vi "AB_820_850_Project_Source_DependencyNode.vi"(6 "dataForPrevious":T2, 7 "action":T1, 8 "error in (no error)":errorcluster, 10 "data in":T6, 11 "buildObject in":T7) -> (0 "error out":errorcluster, 2 "data out":T6, 3 "buildObject out":T7)   [LabVIEW 2020]
doc: "Reads and writes the data to the object property bag."
uses:
  <resource>/Framework/Providers/API/ItemRef.ctl
  <vilib>/AppBuilder/AB_Source_Inclusion.ctl
  <vilib>/AppBuilder/RW_Project/AB_RW_Project_Source_Data_for_Previous.ctl
  <vilib>/AppBuilder/AB_BuildType.ctl
  <vilib>/Utility/lvfile.llb/LVFileType.ctl
  <vilib>/AppBuilder/RW_Project/AB_RW_Project_PropBag_Action.ctl
  <vilib>/Utility/lvfile.llb/NI_FileType.lvlib
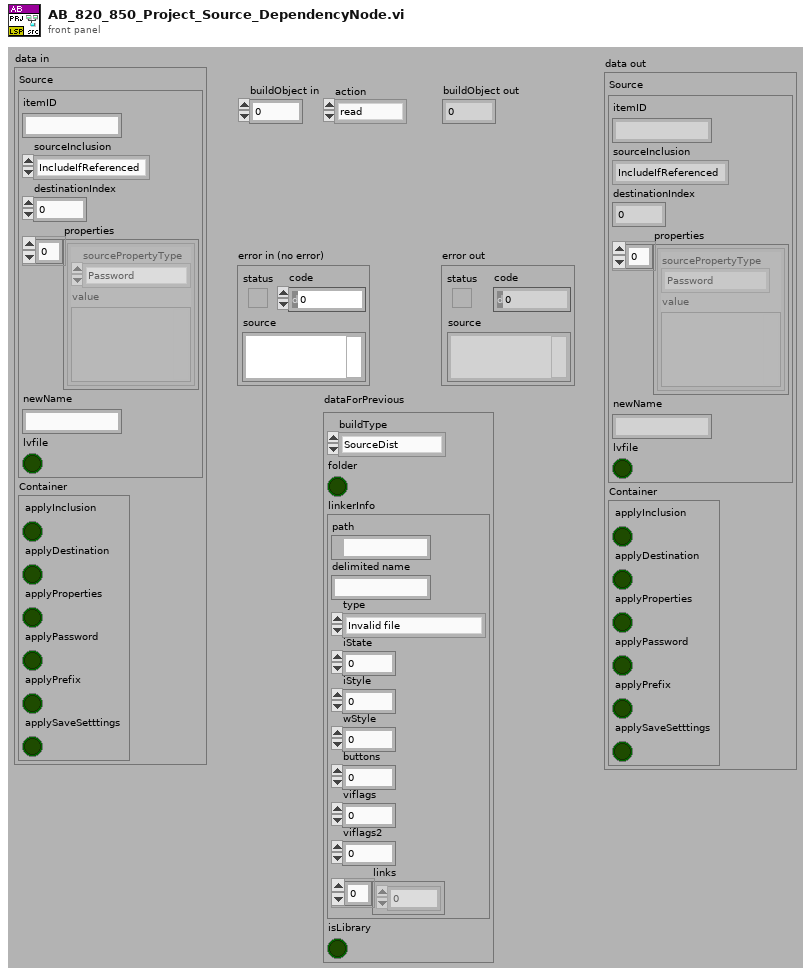
[diagram p1: front panel]
types:
  T1 = typedef "AB_RW_Project_PropBag_Action.ctl" = enum16{"read", "write", "clear", "readPrevious", "writePrevious", "clearPrevious"}
  T2 = typedef "AB_RW_Project_Source_Data_for_Previous.ctl" = cluster{"buildType":T3, "folder":bool, "linkerInfo":cluster{"path":path, "delimited name":string, "type":T4, "iState":u32, "iStyle":u16, "wStyle":u16, "buttons":u16, "viflags":u32, "viflags2":u32, "links":u32[]}, "isLibrary":bool}
  T3 = typedef "AB_BuildType.ctl" = enum16{"SourceDist", "EXE", "DLL", "RTExe"}
  T4 = typedef "NI_FileType.lvlib/LVFileType.ctl" = enum32{"Invalid file", "Unknown type", "Instrument", "Control", "Polymorphic VI", "Project", "Library", "LVClass", "XControl", "XNode", "Shared library", ".NET assembly", "ActiveX interface", "CIN", "Run-time menu", "Palette menu", "Help file", "LLB", "XNode Edit Dependency", "Class Private Data Control", "Statechart", "MathScript .m file", "Ladder Diagram", "LVLibp", "XNode Build Dependency"}
  T5 = typedef "AB_Source_Inclusion.ctl" = enum16{"IncludeIfReferenced", "Include", "Exclude", "TopLevel"}
  T6 = cluster{"Source":cluster{"itemID":string, "sourceInclusion":T5, "destinationIndex":i32, "properties":cluster{"sourcePropertyType":enum16{"Remove block diagram", "Remove front panel", "Password", "Window has title bar", "Show menu bar", "Show vertical scroll bar", "Show horizontal scroll bar", "Show toolbar", "Show Abort button", "Show fp when called", "Window behavior", "Allow user to close window", "Window run-time position", "Run when opened", "Allow debugging", "Auto error handling"}, "value":variant}[], "newName":string, "lvfile":bool}, "Container":cluster{"applyInclusion":bool, "applyDestination":bool, "applyProperties":bool, "applyPassword":bool, "applyPrefix":bool, "applySaveSetttings":bool}}
  T7 = typedef "ItemRef.ctl" = u64
  T8 = cluster{"sourcePropertyType":enum16{"Remove block diagram", "Remove front panel", "Password", "Window has title bar", "Show menu bar", "Show vertical scroll bar", "Show horizontal scroll bar", "Show toolbar", "Show Abort button", "Show fp when called", "Window behavior", "Allow user to close window", "Window run-time position", "Run when opened", "Allow debugging", "Auto error handling"}, "value":variant}
  T9 = enum16{"Remove block diagram", "Remove front panel", "Password", "Window has title bar", "Show menu bar", "Show vertical scroll bar", "Show horizontal scroll bar", "Show toolbar", "Show Abort button", "Show fp when called", "Window behavior", "Allow user to close window", "Window run-time position", "Run when opened", "Allow debugging", "Auto error handling"}
  T10 = cluster{"pre-2010 typedef (disconnected)":enum16{"Remove block diagram", "Remove front panel", "Password", "Window has title bar", "Show menu bar", "Show vertical scroll bar", "Show horizontal scroll bar", "Show toolbar", "Show Abort button", "Show fp when called", "Window behavior", "Allow user to close window", "Window run-time position", "Run when opened", "Allow debugging", "Auto error handling"}, "Value":string}
  T11 = cluster{"sourcePropertyType":enum16{"Remove block diagram", "Remove front panel", "Password", "Window has title bar", "Show menu bar", "Show vertical scroll bar", "Show horizontal scroll bar", "Show toolbar", "Show Abort button", "Show fp when called", "Window behavior", "Allow user to close window", "Window run-time position", "Run when opened", "Allow debugging", "Auto error handling"}, "value":variant}[]
  T12 = cluster{"pre-2010 typedef (disconnected)":enum16{"Remove block diagram", "Remove front panel", "Password", "Window has title bar", "Show menu bar", "Show vertical scroll bar", "Show horizontal scroll bar", "Show toolbar", "Show Abort button", "Show fp when called", "Window behavior", "Allow user to close window", "Window run-time position", "Run when opened", "Allow debugging", "Auto error handling"}, string}
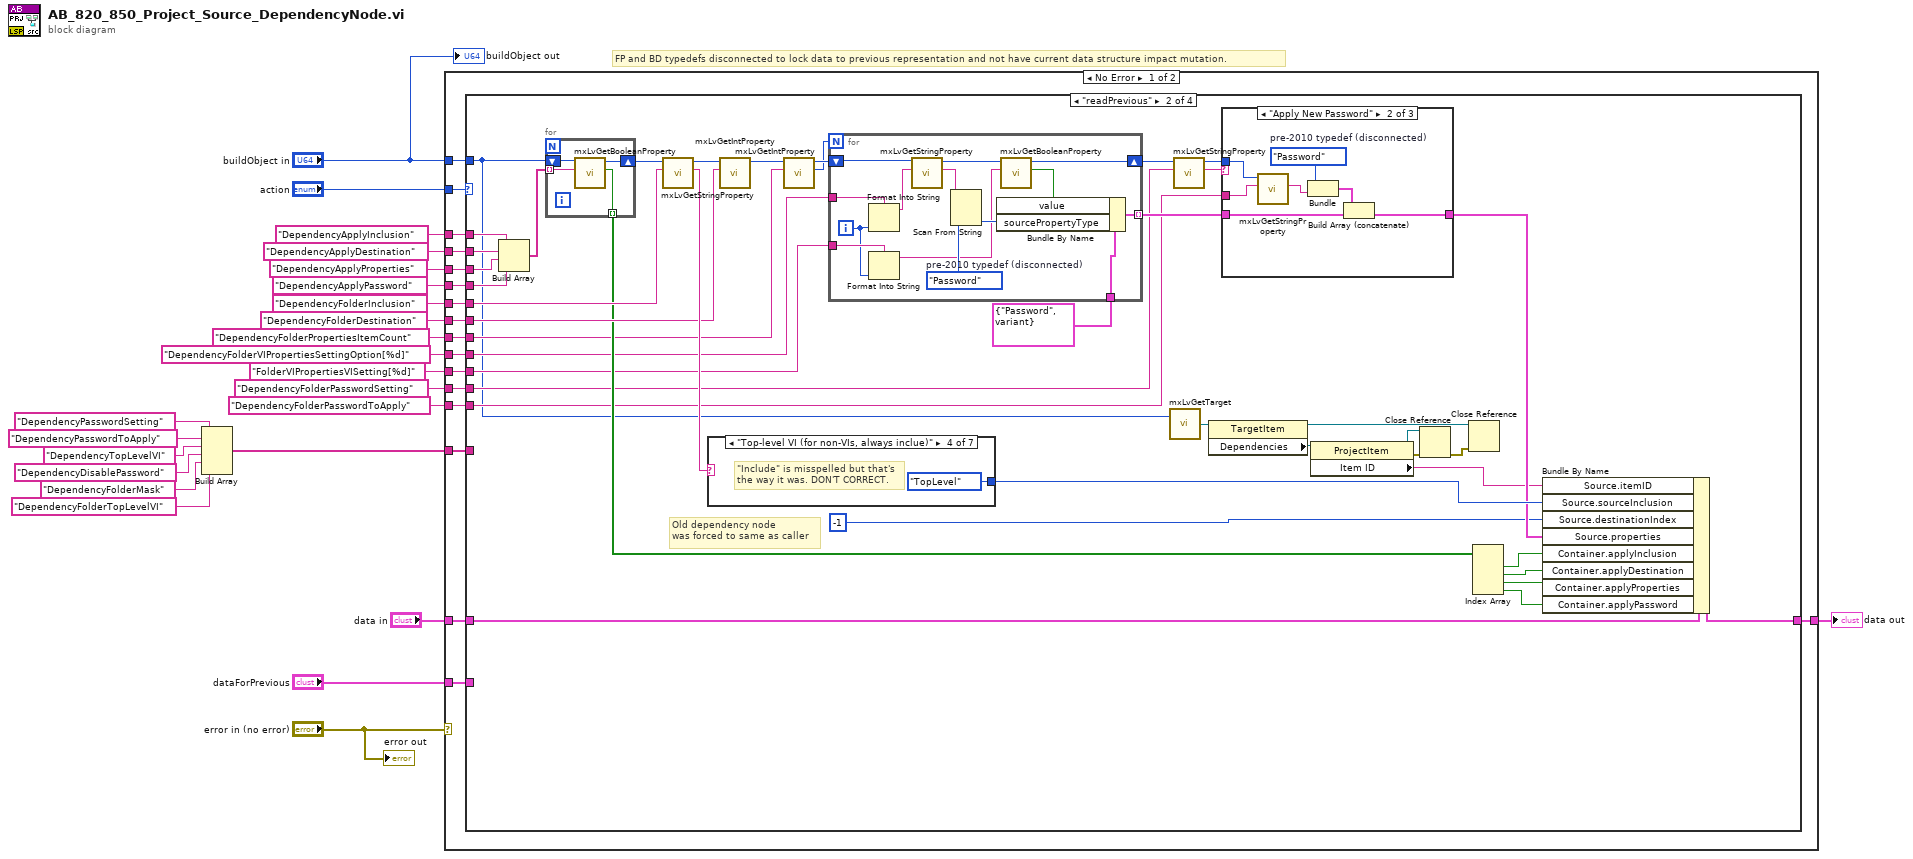
[diagram p0: block diagram]
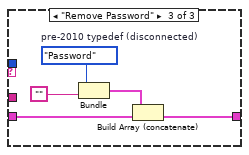
[diagram p4: hidden frame]
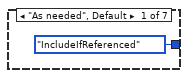
[diagram p5: hidden frame]
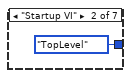
[diagram p6: hidden frame]
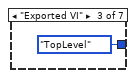
[diagram p7: hidden frame]
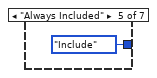
[diagram p8: hidden frame]
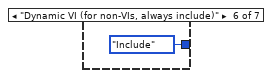
[diagram p9: hidden frame]
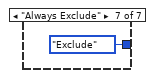
[diagram p10: hidden frame]
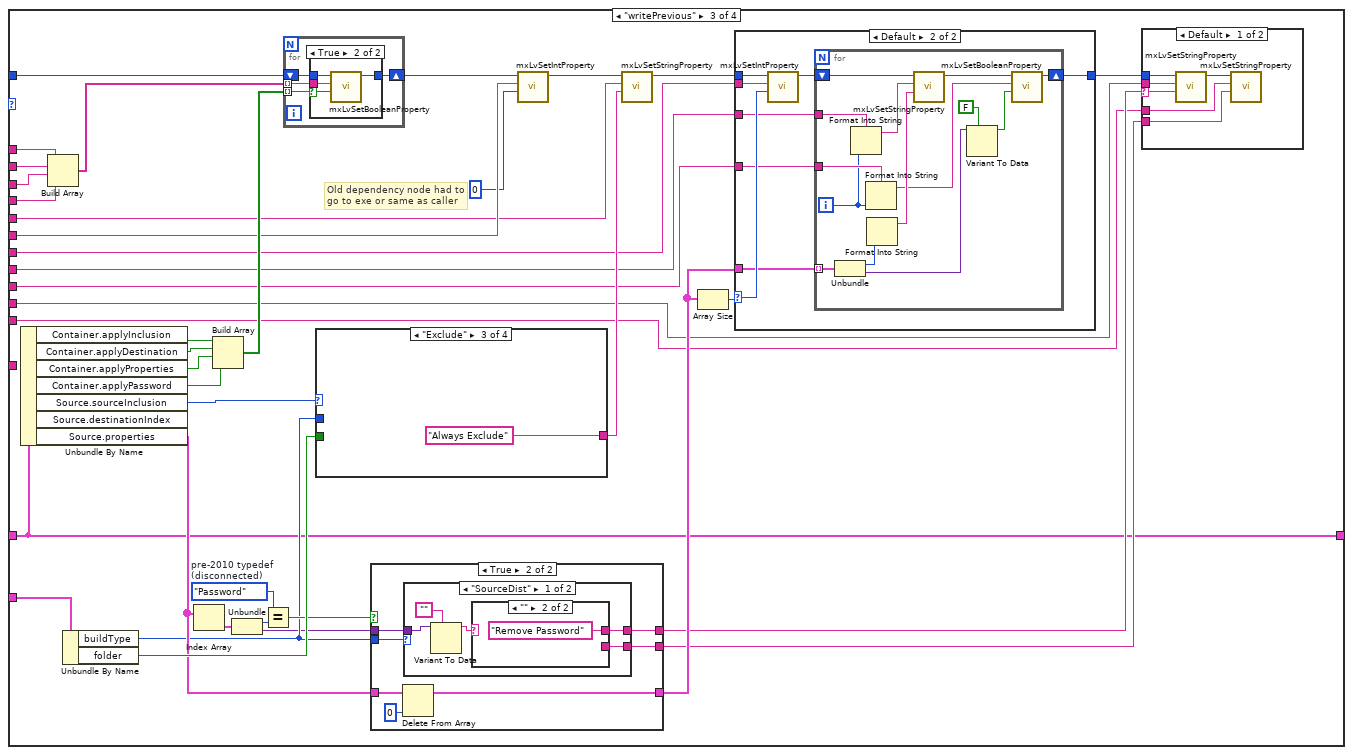
[diagram p11: hidden frame]
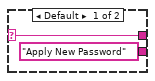
[diagram p15: hidden frame]
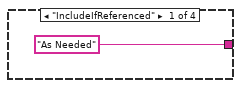
[diagram p17: hidden frame]
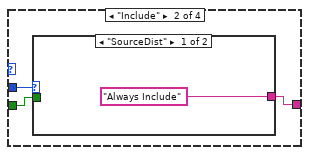
[diagram p18: hidden frame]
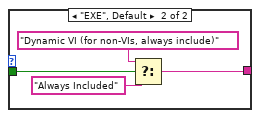
[diagram p19: hidden frame]
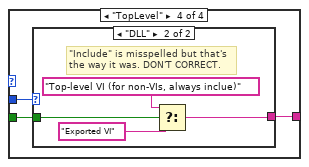
[diagram p20: hidden frame]
diagram:
  # "FP and BD typedefs disconnected to lock data to previous representation and not have current data structure impact mutation."
  n1 = Build Array("DependencyPasswordSetting", "DependencyPasswordToApply", "DependencyTopLevelVI", "DependencyDisablePassword", "DependencyFolderMask", "DependencyFolderTopLevelVI") -> (w2:string[])
  n2 = case shown="No Error" "error in (no error)" {
    tunnel: "buildObject in" -> [w28 _]
    tunnel: "DependencyApplyInclusion" -> [w37 _]
    tunnel: "DependencyFolderInclusion" -> [w41 _]
    tunnel: "DependencyApplyDestination" -> [w38 _]
    tunnel: "DependencyFolderDestination" -> [w40 _]
    tunnel: "DependencyFolderPropertiesItemCount" -> [w34 _]
    tunnel: "DependencyApplyProperties" -> [w36 _]
    tunnel: "data in" -> [w39 w264]
    tunnel: "DependencyApplyPassword" -> [w35 _]
    tunnel: "DependencyFolderVIPropertiesSettingOption[%d]" -> [w33 _]
    tunnel: "FolderVIPropertiesVISetting[%d]" -> [w32 _]
    tunnel: "DependencyFolderPasswordToApply" -> [w31 _]
    tunnel: "DependencyFolderPasswordSetting" -> [w30 _]
    tunnel: [w29 w264] -> w11
    tunnel: "action" -> [w27 _]
    tunnel: "dataForPrevious" -> [w26 _]
    tunnel: w2 -> [w25 _]
    frame No Error {
      n3 = case shown="\"readPrevious\"" w27 {
        tunnel: w41 -> [_ w81 w129 w248]
        tunnel: w40 -> [_ w80 w130 w247]
        tunnel: w39 -> [w42 w79 w123 w253]
        tunnel: w38 -> [_ w78 w140 w251]
        tunnel: w37 -> [_ w77 w141 w252]
        tunnel: w36 -> [_ w76 w139 w250]
        tunnel: w35 -> [_ w75 w138 w249]
        tunnel: w34 -> [_ w58 w128 w244]
        tunnel: w33 -> [_ w57 w127 w242]
        tunnel: w32 -> [_ w56 w126 w241]
        tunnel: w31 -> [_ w55 w124 w239]
        tunnel: w30 -> [_ w54 w125 w240]
        tunnel: [w42 w52 w123 w253] -> w29
        tunnel: w28 -> [_ w51 w142 w246]
        tunnel: w26 -> [_ _ w132 _]
        tunnel: w25 -> [_ _ _ w236]
        frame Default {
        }
        frame "readPrevious" {
          # "Old dependency node\nwas forced to same as caller"
          n4 = Build Array(w77, w78, w76, w75) -> (w74:string[])
          n5 = for {
            tunnel: w74 -> [w112] mode=indexing
            shift-right: [w114] -> w83
            shift-left: w51 -> [w113]
            tunnel: [w111] -> w73 mode=indexing
            n6 = call <resource>:"mxLvGetBooleanProperty.vi"("Tag"=w112, "Item"=w113) -> ("Value"=w111:bool, "Item"=w114:T7)  [unwired: 1 in, 7 out]
          }
          n7 = call <resource>:"mxLvGetStringProperty.vi"("Tag"=w81, "Item"=w83) -> ("Value"=w82:string, "Item"=w68:T7)  [unwired: 1 in, 7 out]
          n8 = case shown="\"Top-level VI (for non-VIs, always inclue)\"" w82 {
            tunnel: [AB_Source_Inclusion."IncludeIfReferenced" ("sourceInfo.sourceInclusion") AB_Source_Inclusion."TopLevel" ("sourceInfo.sourceInclusion") AB_Source_Inclusion."TopLevel" ("sourceInfo.sourceInclusion") AB_Source_Inclusion."TopLevel" ("sourceInfo.sourceInclusion") AB_Source_Inclusion."Include" ("sourceInfo.sourceInclusion") AB_Source_Inclusion."Include" ("sourceInfo.sourceInclusion") AB_Source_Inclusion."Exclude" ("sourceInfo.sourceInclusion")] -> w67
            frame "As needed", Default {
            }
            frame "Startup VI" {
            }
            frame "Exported VI" {
            }
            frame "Top-level VI (for non-VIs, always inclue)" {
              # "\"Include\" is misspelled but that's the way it was. DON'T CORRECT."
            }
            frame "Always Included" {
            }
            frame "Dynamic VI (for non-VIs, always include)" {
            }
            frame "Always Exclude" {
            }
          }
          n9 = call <resource>:"mxLvGetIntProperty.vi"("Tag"=w80, "Item"=w68) -> ("Item"=w59:T7)  [unwired: 1 in, 8 out]
          n10 = call <resource>:"mxLvGetIntProperty.vi"("Tag"=w58, "Item"=w59) -> ("Value"=w60:i32, "Item"=w66:T7)  [unwired: 1 in, 7 out]
          n11 = for {
            N: w60 -> [_]
            tunnel: T8 {"sourcePropertyType"=enum."Password", "value"=variant} ("fileProperties") -> [w108]
            tunnel: [w107] -> w65 mode=indexing
            tunnel: w57 -> [w101]
            tunnel: w56 -> [w98]
            shift-right: [w102] -> w62
            shift-left: w66 -> [w110]
            i -> [w97]
            w104 = T9."Password"  # pre-2010 typedef (disconnected)
            n12 = Format Into String(format string=w101, w97) -> (resulting string=w100:string)  [unwired: 2 in, 1 out]
            n13 = Format Into String(format string=w98, w97) -> (resulting string=w99:string)  [unwired: 2 in, 1 out]
            n14 = call <resource>:"mxLvGetStringProperty.vi"("Tag"=w100, "Item"=w110) -> ("Value"=w105:string, "Item"=w109:T7)  [unwired: 1 in, 7 out]
            n15 = Scan From String(input string=w105, default 1=w104) -> (output 1=w103:T9)  [unwired: 3 in, 3 out]
            n16 = call <resource>:"mxLvGetBooleanProperty.vi"("Tag"=w99, "Item"=w109) -> ("Value"=w106:bool, "Item"=w102:T7)  [unwired: 1 in, 7 out]
            n17 = Bundle By Name(cluster=w108, "value"=w106, "sourcePropertyType"=w103) -> (w107:T8)
          }
          n18 = call <resource>:"mxLvGetTarget.vi"("Item"=w51) -> ("Target"=w50:refnum<vi>)  [unwired: 1 in, 2 out]
          n19 = call <resource>:"mxLvGetStringProperty.vi"("Tag"=w54, "Item"=w62) -> ("Value"=w63:string, "Item"=w64:T7)  [unwired: 1 in, 7 out]
          n20 = property class="TargetItem"(reference=w50) -> (reference out=w43:refnum<vi>, "Dependencies"=w49:refnum<vi>)  [unwired: 1 in, 1 out]
          n21 = case shown="\"Apply New Password\"" w63 {
            tunnel: w64 -> [_ w91 _]
            tunnel: w55 -> [_ w90 _]
            tunnel: w65 -> [w84 w89 w96]
            tunnel: [w84 w85 w93] -> w53
            frame "No Password Change", Default {
            }
            frame "Apply New Password" {
              w88 = T9."Password"  # pre-2010 typedef (disconnected)
              n22 = call <resource>:"mxLvGetStringProperty.vi"("Tag"=w90, "Item"=w91) -> ("Value"=w87:string)  [unwired: 1 in, 8 out]
              n23 = Bundle("pre-2010 typedef (disconnected)"=w88, "Value"=w87) -> (w86:T10)  [unwired: 1 out]
              n24 = Build Array (concatenate)(w86, w89) -> (w85:T11)
            }
            frame "Remove Password" {
              w95 = T9."Password"  # pre-2010 typedef (disconnected)
              n25 = Bundle("pre-2010 typedef (disconnected)"=w95, "") -> (w94:T12)  [unwired: 1 out]
              n26 = Build Array (concatenate)(w94, w96) -> (w93:T11)
            }
          }
          n27 = property class="ProjectItem"(reference=w49) -> (reference out=w46:refnum<vi>, error out=w45:errorcluster, "Item ID"=w48:string)  [unwired: 1 in]
          n28 = Close Reference(reference=w46, error in (no error)=w45) -> (error out=w44:errorcluster)
          n29 = Close Reference(reference=w43, error in (no error)=w44) -> ()  [unwired: 1 out]
          n30 = Index Array(array=w73) -> (element #1=w72:bool, element #2=w71:bool, element #3=w70:bool, element #4=w69:bool)  [unwired: 4 in]
          n31 = Bundle By Name(cluster=w79, "Source.itemID"=w48, "Source.sourceInclusion"=w67, "Source.destinationIndex"=-1, "Source.properties"=w53, "Container.applyInclusion"=w72, "Container.applyDestination"=w71, "Container.applyProperties"=w70, "Container.applyPassword"=w69) -> (w52:T6)
        }
        frame "writePrevious" {
          w154 = T9."Password"  # pre-2010 typedef (disconnected)
          # "Old dependency node had to go to exe or same as caller"
          n32 = Unbundle By Name(w123) -> ("Container.applyInclusion"=w137:bool, "Container.applyDestination"=w136:bool, "Container.applyProperties"=w135:bool, "Container.applyPassword"=w134:bool, "Source.sourceInclusion"=w159:T5, "Source.properties"=w152:T11)  [unwired: 1 out]
          n33 = Build Array(w141, w140, w139, w138) -> (w143:string[])
          n34 = Unbundle By Name(w132) -> ("buildType"=w151:T3, "folder"=w158:bool)
          n35 = Index Array(array=w152) -> (element=w156:T8)  [unwired: 1 in]
          n36 = Build Array(w137, w136, w135, w134) -> (w133:bool[])
          n37 = Unbundle(w156) -> ("sourcePropertyType"=w155:T9, "value"=w150:variant)
          n38 = Equal?(x=w154, y=w155) -> (x = y?=w153:bool)
          n39 = for {
            tunnel: w143 -> [w162] mode=indexing
            shift-right: [w163] -> w131
            shift-left: w142 -> [w164]
            tunnel: w133 -> [w161] mode=indexing
            n40 = case shown="True" w161 {
              selector: w161 -> [_ w166]
              tunnel: w164 -> [w165 w169]
              tunnel: [w165 w168] -> w163
              tunnel: w162 -> [_ w167]
              frame False {
              }
              frame True {
                n41 = call <resource>:"mxLvSetBooleanProperty.vi"("Value (F)"=w166, "Tag"=w167, "Item"=w169) -> ("Item"=w168:T7)  [unwired: 2 in, 6 out]
              }
            }
          }
          n42 = case shown="\"Exclude\"" w159 {
            tunnel: w151 -> [_ w195 _ w204]
            tunnel: w158 -> [_ w194 _ w203]
            tunnel: ["As Needed" w193 "Always Exclude" w202] -> w157
            frame "IncludeIfReferenced" {
            }
            frame "Include" {
              n43 = case shown="\"SourceDist\"" w195 {
                tunnel: w194 -> [_ w200]
                tunnel: ["Always Include" w197] -> w193
                frame "SourceDist" {
                }
                frame "EXE", Default {
                  n44 = Select(t="Dynamic VI (for non-VIs, always include)", s=w200, f="Always Included") -> (s? t:f=w197:string)
                }
              }
            }
            frame "Exclude" {
            }
            frame "TopLevel" {
              n45 = case shown="\"DLL\"" w204 {
                tunnel: w203 -> [w208 w212]
                tunnel: [w205 w209] -> w202
                frame "EXE", Default {
                  # "\"Include\" is misspelled but that's the way it was. DON'T CORRECT."
                  n46 = Select(t="Top-level VI (for non-VIs, always inclue)", s=w208, f="Startup VI") -> (s? t:f=w205:string)
                }
                frame "DLL" {
                  # "\"Include\" is misspelled but that's the way it was. DON'T CORRECT."
                  n47 = Select(t="Top-level VI (for non-VIs, always inclue)", s=w212, f="Exported VI") -> (s? t:f=w209:string)
                }
              }
            }
          }
          n48 = case shown="True" w153 {
            tunnel: w152 -> [w176 w183]
            tunnel: [w176 w181] -> w149
            tunnel: w151 -> [_ w180]
            tunnel: w150 -> [_ w179]
            tunnel: [_ w178] -> w146
            tunnel: [_ w177] -> w144
            frame False {
            }
            frame True {
              n49 = Delete From Array(array=w183, index=0) -> (array with subset deleted=w181:T11)  [unwired: 1 in, 1 out]
              n50 = case shown="\"SourceDist\"" w180 {
                tunnel: w179 -> [w187 _]
                tunnel: [w185 _] -> w178
                tunnel: [w184 _] -> w177
                frame "SourceDist" {
                  n51 = Variant To Data(type="", Variant=w187) -> (data=w186:string)  [unwired: 1 in, 1 out]
                  n52 = case shown="\"\"" w186 {
                    selector: w186 -> [w190 _]
                    tunnel: [w190 "Remove Password"] -> w185
                    tunnel: ["Apply New Password" _] -> w184
                    frame Default {
                    }
                    frame "" {
                    }
                  }
                }
                frame Default {
                }
              }
            }
          }
          n53 = call <resource>:"mxLvSetIntProperty.vi"("Value (0)"=0, "Tag"=w130, "Item"=w131) -> ("Item"=w148:T7)  [unwired: 2 in, 6 out]
          n54 = call <resource>:"mxLvSetStringProperty.vi"("Value (\"\")"=w157, "Tag"=w129, "Item"=w148) -> ("Item"=w147:T7)  [unwired: 2 in, 6 out]
          n55 = Array Size(array=w149) -> (size(s)=w160:i32)
          n56 = case shown="Default" w160 {
            selector: w160 -> [_ w219]
            tunnel: w149 -> [_ w217]
            tunnel: w128 -> [_ w221]
            tunnel: w147 -> [w213 w220]
            tunnel: w127 -> [_ w216]
            tunnel: w126 -> [_ w215]
            tunnel: [w213 w214] -> w145
            frame 0 {
            }
            frame Default {
              n57 = call <resource>:"mxLvSetIntProperty.vi"("Value (0)"=w219, "Tag"=w221, "Item"=w220) -> ("Item"=w218:T7)  [unwired: 2 in, 6 out]
              n58 = for {
                shift-right: [w226] -> w214
                shift-left: w218 -> [w235]
                tunnel: w217 -> [w234] mode=indexing
                tunnel: w216 -> [w233]
                tunnel: w215 -> [w230]
                i -> [w229]
                n59 = Unbundle(w234) -> ("sourcePropertyType"=w228:T9, "value"=w224:variant)
                n60 = Format Into String(format string=w233, w229) -> (resulting string=w232:string)  [unwired: 2 in, 1 out]
                n61 = Format Into String(format string=w230, w229) -> (resulting string=w225:string)  [unwired: 2 in, 1 out]
                n62 = Format Into String(w228) -> (resulting string=w231:string)  [unwired: 3 in, 1 out]
                n63 = call <resource>:"mxLvSetStringProperty.vi"("Value (\"\")"=w231, "Tag"=w232, "Item"=w235) -> ("Item"=w227:T7)  [unwired: 2 in, 6 out]
                n64 = Variant To Data(type=FALSE, Variant=w224) -> (data=w222:bool)  [unwired: 1 in, 1 out]
                n65 = call <resource>:"mxLvSetBooleanProperty.vi"("Value (F)"=w222, "Tag"=w225, "Item"=w227) -> ("Item"=w226:T7)  [unwired: 2 in, 6 out]
              }
            }
          }
          n66 = case shown="Default" w146 {
            selector: w146 -> [w173 _]
            tunnel: w145 -> [w175 _]
            tunnel: w125 -> [w174 _]
            tunnel: w144 -> [w171 _]
            tunnel: w124 -> [w170 _]
            frame Default {
              n67 = call <resource>:"mxLvSetStringProperty.vi"("Value (\"\")"=w173, "Tag"=w174, "Item"=w175) -> ("Item"=w172:T7)  [unwired: 2 in, 6 out]
              n68 = call <resource>:"mxLvSetStringProperty.vi"("Value (\"\")"=w171, "Tag"=w170, "Item"=w172) -> ()  [unwired: 2 in, 7 out]
            }
            frame "" {
            }
          }
        }
        frame "clearPrevious" {
          n69 = Build Array (concatenate)(w252, w251, w250, w249, w248, w247, w244, w240, w239, w236) -> (w237:string[])
          n70 = call <resource>:"mxLvGetIntProperty.vi"("Tag"=w244, "Item"=w246) -> ("Value"=w243:i32, "Item"=w245:T7)  [unwired: 1 in, 7 out]
          n71 = for {
            N: w243 -> [_]
            tunnel: w242 -> [w263]
            shift-right: [w258] -> w238
            shift-left: w245 -> [w260]
            tunnel: w241 -> [w261]
            i -> [w262]
            n72 = Format Into String(format string=w263, w262) -> (resulting string=w257:string)  [unwired: 2 in, 1 out]
            n73 = call <resource>:"mxLvDeleteProperty.vi"("Tag"=w257, "Item"=w260) -> ("Item"=w259:T7)  [unwired: 1 in, 8 out]
            n74 = Format Into String(format string=w261, w262) -> (resulting string=w256:string)  [unwired: 2 in, 1 out]
            n75 = call <resource>:"mxLvDeleteProperty.vi"("Tag"=w256, "Item"=w259) -> ("Item"=w258:T7)  [unwired: 1 in, 8 out]
          }
          n76 = for {
            tunnel: w238 -> [w255]
            tunnel: w237 -> [w254] mode=indexing
            n77 = call <resource>:"mxLvDeleteProperty.vi"("Tag"=w254, "Item"=w255) -> ()  [unwired: 1 in, 9 out]
          }
        }
      }
    }
    frame Error {
    }
  }
  "data out" <- w11
  "error out" <- "error in (no error)"
  "buildObject out" <- "buildObject in"
